vi "LJ-T7 MX.vi"() -> ()   [LabVIEW 2015]
uses:
  T7 Stream Config KAG.ctl
  T7 IP Config KAG.ctl
  <vilib>/Analysis/5stat.llb/RMS (DBL).vi
  <vilib>/Utility/file.llb/Write Delimited Spreadsheet (DBL).vi
  T7 Stream Globals KAG.vi
  <vilib>/Analysis/NI_AALPro.lvlib
  <vilib>/Analysis/NI_AALBase.lvlib
panel:
  in  "Tab Control":enum32{"Setup", "Statistics"}(tab)
  in  "Strm Config in":T1={"Scan Rate (Hz)"=1024.0, "Samples Per Packet"=512, "Resolution Index"=0, "Buffer Size (bytes)"=32768, "NumScans"=512, "Read Timeout (ms)"=5000, "Scan Table"=[{"Channel"=4, "BipGain"=0, "Input Config"="Differential"}, {"Channel"=6, "BipGain"=0, "Input Config"="Differential"}, {"Channel"=8, "BipGain"=0, "Input Config"="Differential"}, {"Channel"=10, "BipGain"=0, "Input Config"="Differential"}]} {"Samples Per Packet" max=512 step=1; "Buffer Size (bytes)" max=32768 step=1; "Resolution Index" max=8 step=1; "Scan Rate (Hz)" max=100000; "Scan Table"."BipGain" items=["x1", "x10", "x100", "x1000"]; "Scan Table"."Channel" step=1}
  in  "IP Config in":T2={"Connection ID In"=refnum, "Connection ID Out"=refnum, "Device IP"="192.168.126.147", "Port"=502}
  in  "Log Path":path=path "/Macintosh HD/Users/kgompertz/Desktop/untitled"
  in  "Log Data":bool
  in  "Append?":bool=TRUE
  out "AIN#":u32[](array[numeric])
  out "Variance":dbl[](array[numeric]) format="%_4g"
  out "Std Dev":dbl[](array[numeric]) format="%.4f"
  out "Mean":dbl[](array[numeric]) format="%.4f"
  out "RMS":dbl[](array[numeric]) format="%.4f"
  out "error out":errorcluster
  out "Startup":bool
  out "Strm Config out":T1={"Scan Rate (Hz)"=1000.0, "Samples Per Packet"=512, "Resolution Index"=0, "Buffer Size (bytes)"=32768, "NumScans"=1500, "Read Timeout (ms)"=5000, "Scan Table"=[{"Channel"=0, "BipGain"=0, "Input Config"="Single-Ended"}, {"Channel"=1, "BipGain"=0, "Input Config"="Single-Ended"}, {"Channel"=2, "BipGain"=0, "Input Config"="Single-Ended"}, {"Channel"=3, "BipGain"=0, "Input Config"="Single-Ended"}]} {"Samples Per Packet" max=512 step=1; "Buffer Size (bytes)" max=32768 step=1; "Resolution Index" max=8 step=1; "Scan Rate (Hz)" max=100000; "Scan Table"."BipGain" items=["x1", "x10", "x100", "x1000"]; "Scan Table"."Channel" step=1}
  out "IP Config out":T3={"Connection ID In"=refnum, "Connection ID Out"=refnum, "Device IP"="", "Port"=502}
  out "Current Block #":i32
  in  "Stop Button":bool
  out "Waveform Graph":dbl[][](graph)
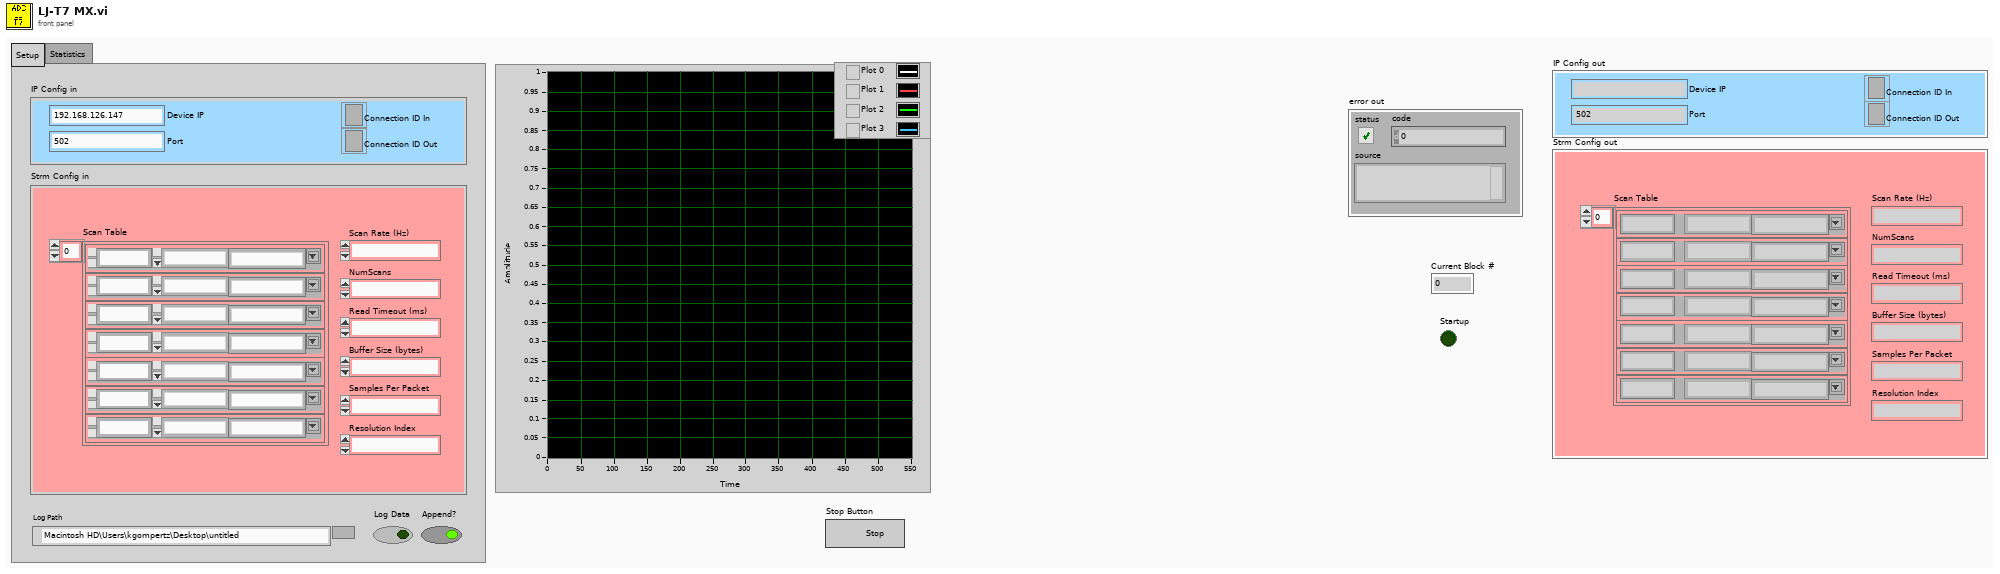
[diagram p1: front panel]
types:
  T1 = typedef "T7 Stream Config KAG.ctl" = cluster{"Scan Rate (Hz)":sgl, "Samples Per Packet":u32, "Resolution Index":u32, "Buffer Size (bytes)":u32, "NumScans":u32, "Read Timeout (ms)":u32, "Scan Table":cluster{"Channel":u32, "BipGain":u32, "Input Config":string}[]}
  T2 = typedef "T7 IP Config KAG.ctl" = cluster{"Connection ID In":refnum<k5>, "Connection ID Out":refnum<k5>, "Device IP":string, "Port":i32}
  T3 = cluster{"Connection ID In":refnum<k5>, "Connection ID Out":refnum<k5>, "Device IP":string, "Port":i32}
  T4 = cluster{"Channel":u32, "BipGain":u32, "Input Config":string}[]
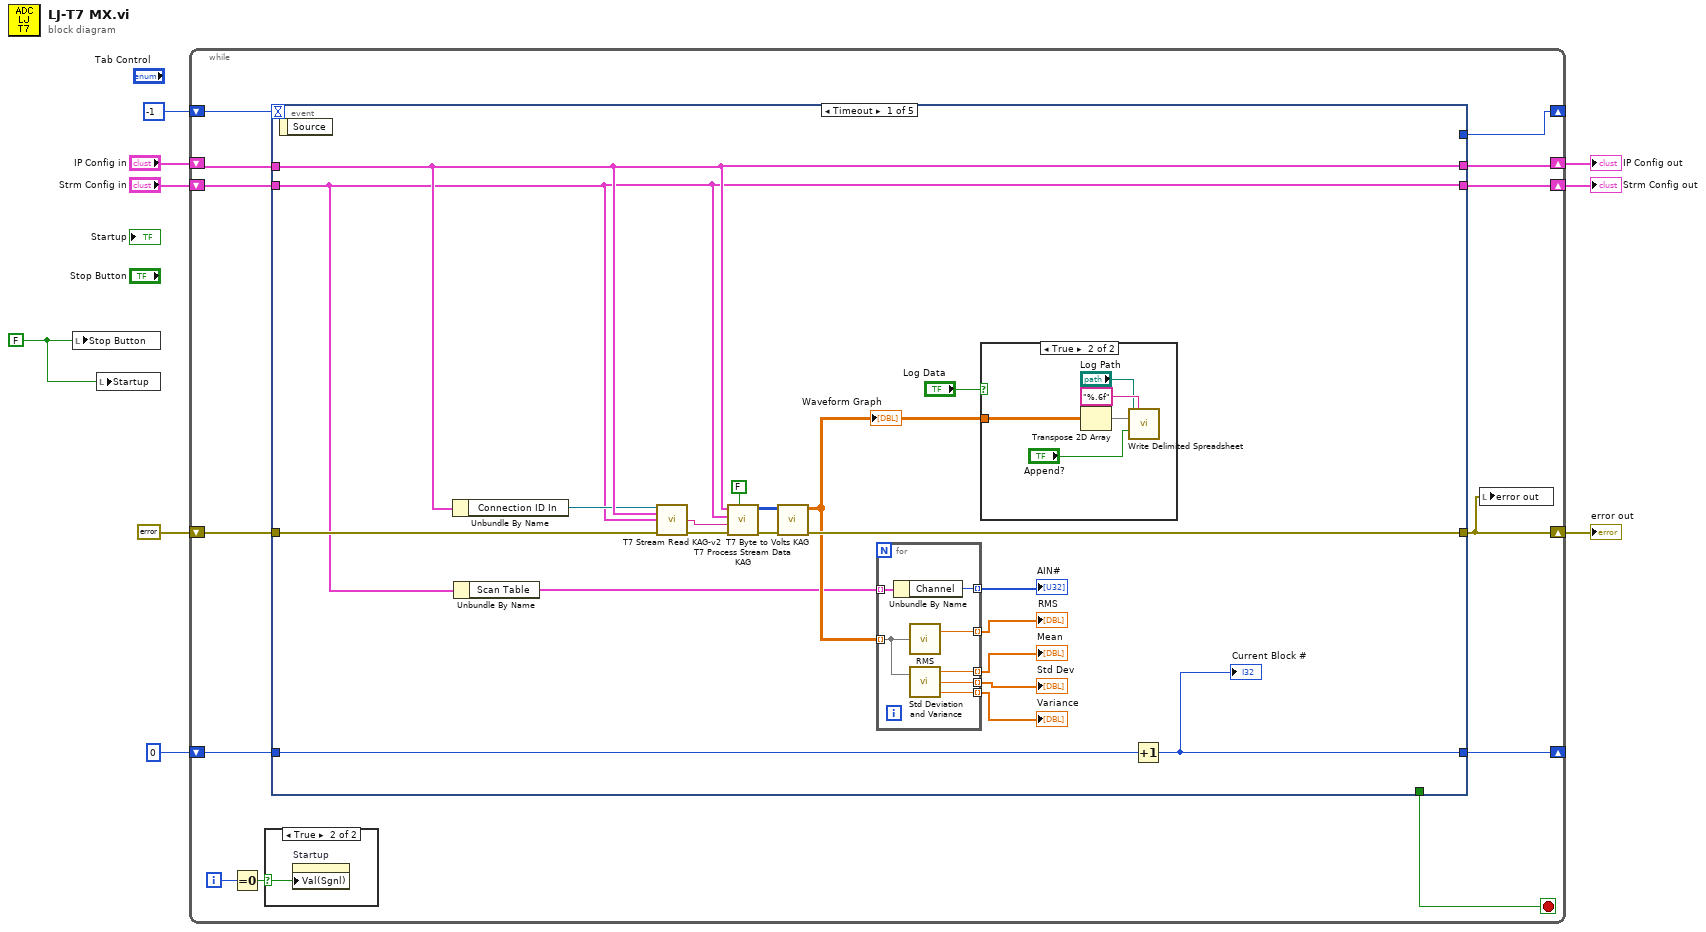
[diagram p0: block diagram]
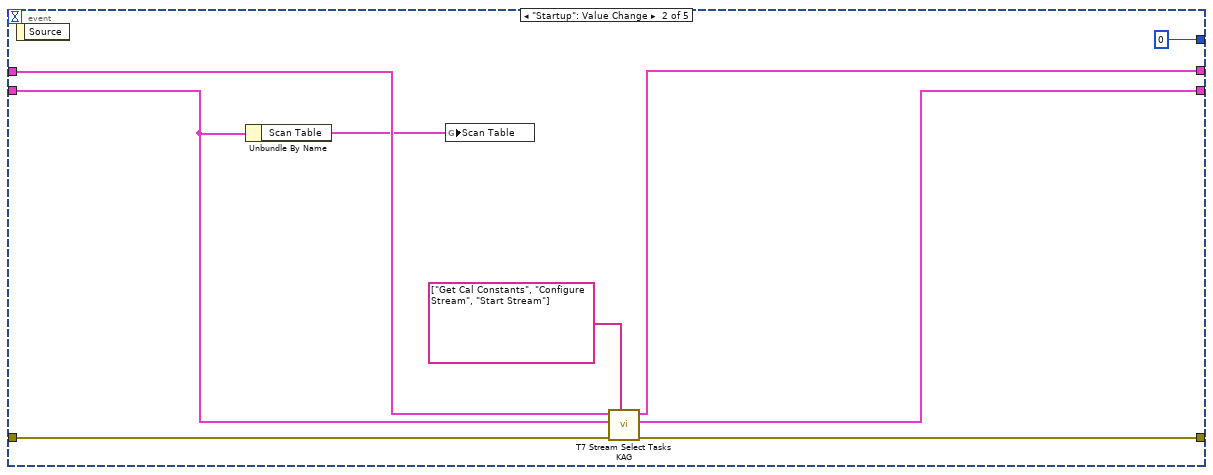
[diagram p4: hidden frame]
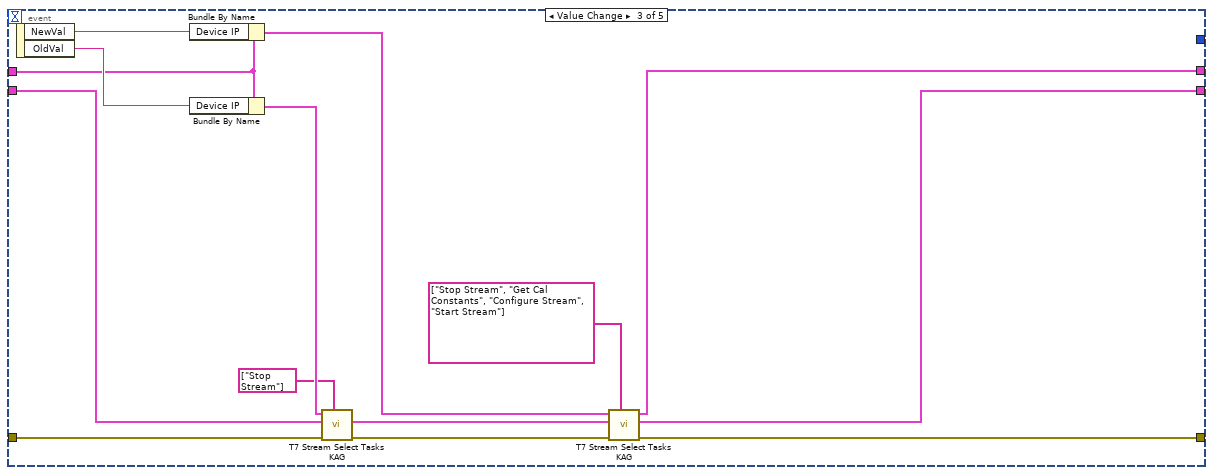
[diagram p5: hidden frame]
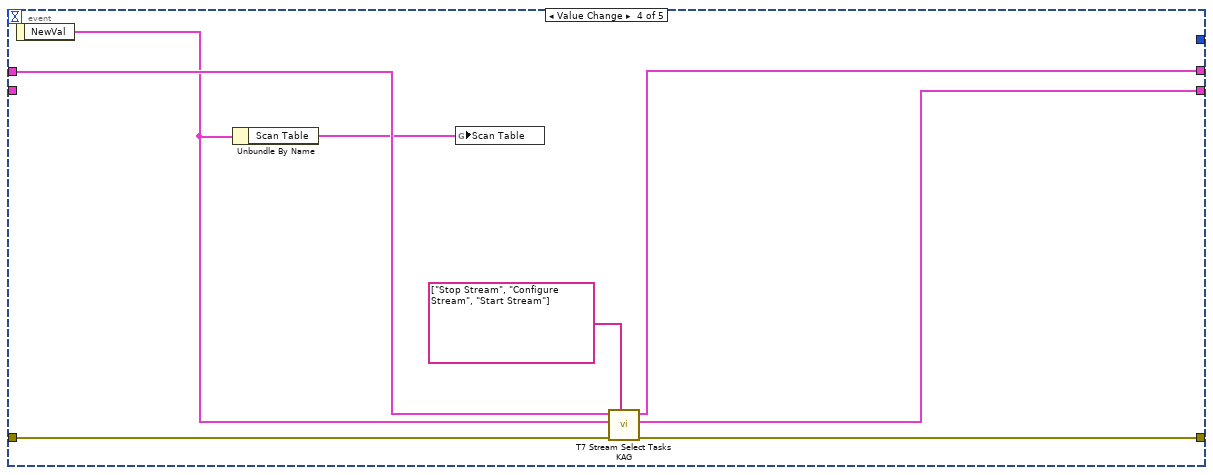
[diagram p6: hidden frame]
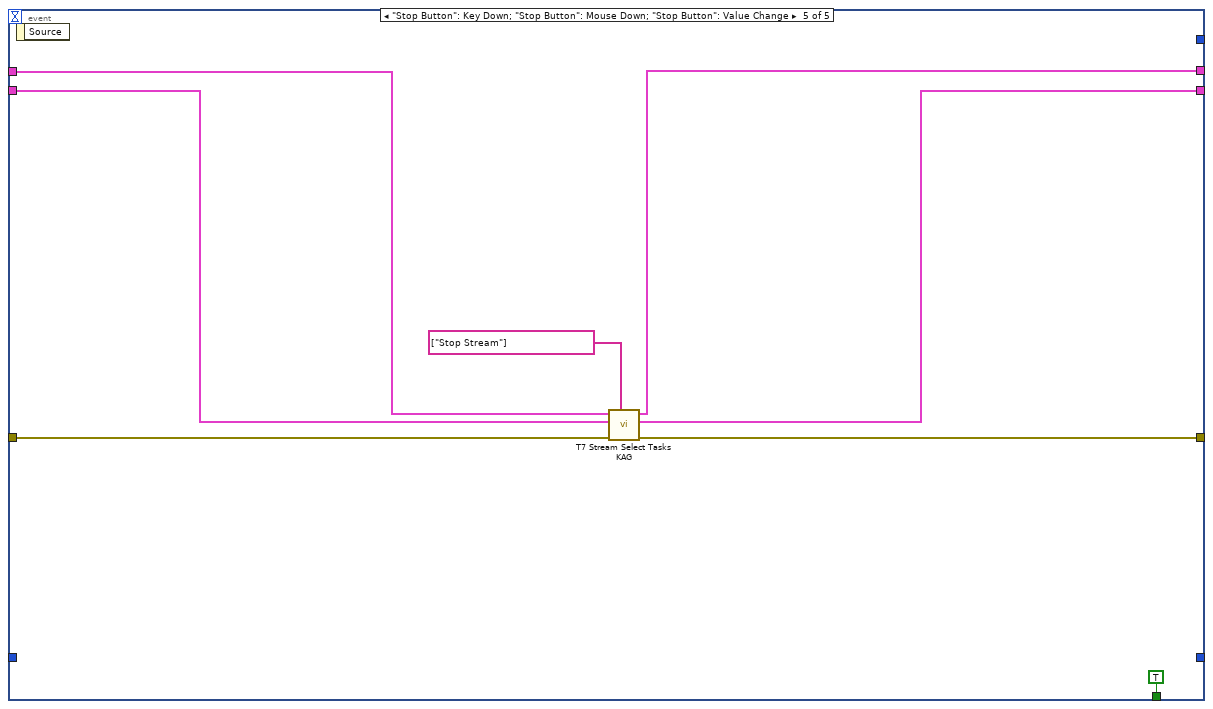
[diagram p7: hidden frame]
diagram:
  w3 = FALSE ("Stop Button")
  n1 = local write "Stop Button"(w3) -> ()
  n2 = local write "Startup"(w3) -> ()
  n3 = while {
    shift-right: [w15] -> w5
    shift-left: "IP Config in" -> [w17]
    shift-right: [w14] -> w4
    shift-left: "Strm Config in" -> [w16]
    shift-right: [w10] -> w2
    shift-left: errorcluster {"status"=FALSE, "code"=0, "source"=""} ("error IO") -> [w13]
    shift-right: [w18] -> _
    shift-left: 0 -> [w19]
    shift-right: [w11] -> _
    shift-left: -1 -> [w12]
    i -> [w22]
    stop <- w20 stop-if-true
    n4 = Equal To 0?(x=w22) -> (x = 0?=w21:bool)
    n5 = case shown="True" w21 {
      selector: w21 -> [_ w23]
      frame False {
      }
      frame True {
        n6 = property on="Startup" class="Bool (strict)"("Val(Sgnl)"=w23) -> ()  [unwired: 2 in, 2 out]
      }
    }
    n7 = event shown="[0] Timeout" {
      selector: _ -> [_ _ _ _ _]
      dyn-events: _ -> [_ _ _ _ _]
      timeout: w12 -> [_ _ _ _ _]
      tunnel: [_ _ _ _ TRUE] -> w20
      tunnel: w19 -> [w35 _ _ _ _]
      tunnel: [w43 _ _ _ _] -> w18
      tunnel: w17 -> [w34 w61 w67 w82 w90]
      tunnel: w16 -> [w29 w57 w70 _ w89]
      tunnel: [w34 w60 w74 w81 w88] -> w15
      tunnel: [w29 w59 w73 w80 w87] -> w14
      tunnel: w13 -> [w37 w63 w76 w84 w92]
      tunnel: [w36 w62 w75 w83 w91] -> w10
      tunnel: [_ 0 _ _ _] -> w11
      event Timeout {
        n8 = event-data() -> ()  [unwired: 1 in, 1 out]
        n9 = Unbundle By Name(w34) -> ("Connection ID In"=w33:refnum<k5>)
        n10 = Unbundle By Name(w29) -> ("Scan Table"=w25:T4)
        n11 = call "T7 Stream Read KAG-v2.vi"("Connection ID In"=w33, "IP Configuration"=w34, "Stream Configuration"=w29, "error in"=w37) -> ("TCP Data"=w32:string, "error out"=w38:errorcluster)  [unwired: 9 in, 1 out]
        n12 = call "T7 Process Stream Data KAG.vi"("Backlog"=FALSE, "error in"=w38, "TCP Data In"=w32, "Stream Configuration"=w29, "IP Configuration"=w34) -> ("error out"=w39:errorcluster, "Data"=w40:u16[][])  [unwired: 3 in, 2 out]
        n13 = call "T7 Byte to Volts KAG.vi"("error in"=w39, "Byte Data"=w40) -> ("error out"=w36:errorcluster, "Float Data"=w31:dbl[][])  [unwired: 8 in]
        "Waveform Graph" <- w31
        n14 = for {
          tunnel: w31 -> [w50] mode=indexing
          tunnel: [w49] -> w30 mode=indexing
          tunnel: [w48] -> w28 mode=indexing
          tunnel: [w47] -> w27 mode=indexing
          tunnel: [w46] -> w26 mode=indexing
          tunnel: w25 -> [w45] mode=indexing
          tunnel: [w44] -> w24 mode=indexing
          n15 = Unbundle By Name(w45) -> ("Channel"=w44:u32)
          n16 = call-poly <vilib>:"RMS.vi"("X"=w50) -> ("rms value"=w49:dbl)  [unwired: 1 out]
          n17 = call <vilib>:"Std Deviation and Variance.vi"("X"=w50) -> ("mean"=w48:dbl, "standard deviation"=w47:dbl, "variance"=w46:dbl)  [unwired: 1 in]
        }
        "RMS" <- w30
        "Variance" <- w26
        "Mean" <- w28
        "Std Dev" <- w27
        "AIN#" <- w24
        n18 = case shown="True" "Log Data" {
          tunnel: w31 -> [_ w53]
          frame False {
          }
          frame True {
            n19 = Transpose 2D Array(2D array=w53) -> (transposed array=w54:dbl[][])
            n20 = call-poly <vilib>:"Write Delimited Spreadsheet.vi"("file path (dialog if empty)"="Log Path", "format (%.3f)"="%.6f", "2D data"=w54, "append to file? (F)"="Append?") -> ()  [unwired: 10 in, 2 out]
          }
        }
        n21 = Increment(x=w35) -> (x+1=w43:i32)
        "Current Block #" <- w43
      }
      event "Startup": Value Change {
        n22 = event-data() -> ()  [unwired: 1 in, 1 out]
        n23 = Unbundle By Name(w57) -> ("Scan Table"=w56:T4)
        n24 = global write "T7 Stream Globals KAG.vi" "Scan Table"(w56) -> ()
        n25 = call "T7 Stream Select Tasks KAG.vi"("Task Selector Array"=string[] ["Get Cal Constants", "Configure Stream", "Start Stream"], "error in"=w63, "Strm Config in"=w57, "IP Config in"=w61) -> ("error out"=w62:errorcluster, "Strm Config out"=w59:T1, "IP Config out"=w60:T3)  [unwired: 5 in]
      }
      event Value Change {
        n26 = event-data() -> ("NewVal"=w72:string, "OldVal"=w68:string)  [unwired: 1 in]
        n27 = Bundle By Name(cluster=w67, "Device IP"=w72) -> (w71:T2)
        n28 = Bundle By Name(cluster=w67, "Device IP"=w68) -> (w66:T2)
        n29 = call "T7 Stream Select Tasks KAG.vi"("Task Selector Array"=string[] ["Stop Stream"], "Strm Config in"=w70, "IP Config in"=w66) -> ("Strm Config out"=w69:T1)  [unwired: 6 in, 2 out]
        n30 = call "T7 Stream Select Tasks KAG.vi"("Task Selector Array"=string[] ["Stop Stream", "Get Cal Constants", "Configure Stream", "Start Stream"], "error in"=w76, "Strm Config in"=w69, "IP Config in"=w71) -> ("error out"=w75:errorcluster, "Strm Config out"=w73:T1, "IP Config out"=w74:T3)  [unwired: 5 in]
      }
      event Value Change {
        n31 = event-data() -> ("NewVal"=w79:T1)  [unwired: 1 in]
        n32 = Unbundle By Name(w79) -> ("Scan Table"=w78:T4)
        n33 = global write "T7 Stream Globals KAG.vi" "Scan Table"(w78) -> ()
        n34 = call "T7 Stream Select Tasks KAG.vi"("Task Selector Array"=string[] ["Stop Stream", "Configure Stream", "Start Stream"], "error in"=w84, "Strm Config in"=w79, "IP Config in"=w82) -> ("error out"=w83:errorcluster, "Strm Config out"=w80:T1, "IP Config out"=w81:T3)  [unwired: 5 in]
      }
      event "Stop Button": Key Down; "Stop Button": Mouse Down; "Stop Button": Value Change {
        n35 = event-data() -> ()  [unwired: 1 in, 1 out]
        n36 = call "T7 Stream Select Tasks KAG.vi"("Task Selector Array"=string[] ["Stop Stream"], "error in"=w92, "Strm Config in"=w89, "IP Config in"=w90) -> ("error out"=w91:errorcluster, "Strm Config out"=w87:T1, "IP Config out"=w88:T3)  [unwired: 5 in]
      }
    }
    n37 = local write "error out"(w10) -> ()
  }
  "IP Config out" <- w5
  "Strm Config out" <- w4
  "error out" <- w2
